vi "Test - Create Property.vi"   [LabVIEW 2020, in "JSON Schema Generator.lvlib"]
uses:
  JSON Schema Generator.lvlib
  <vilib>/addons/_JKI Toolkits/Caraya/classes/Test/Test.lvclass
  <vilib>/Utility/Data Type/Type Definitions/Data Type.ctl
  <vilib>/Utility/Data Type/NI_Data Type.lvlib
  <vilib>/addons/_JKI Toolkits/Caraya/classes/Assert/Assert.lvclass
  <vilib>/JDP Science/JSONtext/JSONtext.lvlib
  <vilib>/addons/_JKI Toolkits/Caraya/classes/Assert/Assert Equal Value_Variant.vi
  f974771b-0b98-47eb-9ce7-aca3fa1358ef.vi
  <vilib>/addons/_JKI Toolkits/Caraya/classes/Assert/Assert Not Error.vi
types:
  T1 = enum16{"Normal Description", "JSON Description"}[]
  T2 = typedef "NI_Data Type.lvlib/Data Type.ctl" = enum8{"Invalid Type", "Void", "I8", "I16", "I32", "I64", "U8", "U16", "U32", "U64", "Single Float", "Double Float", "Extended Float", "Single Complex", "Double Complex", "Extended Complex", "Enum U8", "Enum U16", "Enum U32", "Enum U64", "Single Float With Unit", "Double Float With Unit", "Extended Float With Unit", "Single Complex with Unit", "Double Complex with Unit", "Extended Complex with Unit", "Boolean", "String", "Path", "Picture", "Tag", "Array", "Cluster", "Variant", "LV Variant", "Waveform", "Timestamp", "Digital Waveform", "Digital Data", "ExpressData", "Refnum", "External Data", "VI", "Poly VI", "LabVIEW Class Instance", "Fixed Point", "Set Collection", "Map Collection"}
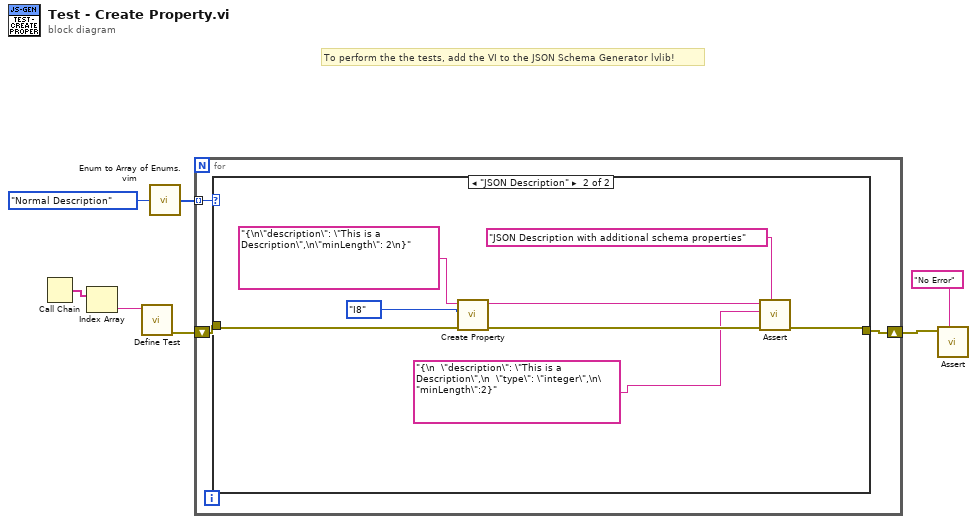
[diagram p0: block diagram]
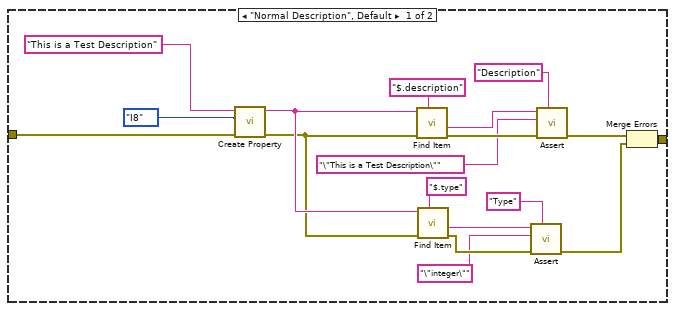
[diagram p2: hidden frame]
diagram:
  # "To perform the the tests, add the VI to the JSON Schema Generator lvlib!"
  n1 = Call Chain() -> (call chain=w7:string[])
  n2 = Index Array(array=w7) -> (element=w6:string)  [unwired: 1 in]
  n3 = call <vilib>:"Define Test.vi"("Label (VI Title)"=w6) -> ("error out"=w5:errorcluster)  [unwired: 9 in, 1 out]
  n4 = call "Enum to Array of Enums.vim"("enum"=enum16{"Normal Description", "JSON Description"}."Normal Description") -> ("array of enums"=w1:T1)
  n5 = for {
    shift-right: [w9] -> w3
    shift-left: w5 -> [w10]
    tunnel: w1 -> [w8] mode=indexing
    n6 = case shown="\"JSON Description\"" w8 {
      tunnel: w10 -> [w28 w32]
      tunnel: [w11 w31] -> w9
      frame "Normal Description", Default {
        n7 = call "Create Property.vi"("error in"=w28, "Labview Type"=Data_Type."I8", "Description"="This is a Test Description") -> ("error out"=w12:errorcluster, "JSON Schema Property out"=w18:string)  [unwired: 7 in]
        n8 = call <vilib>:"Find Item.vi"("$Path or Item Name"="$.description", "error in (no error)"=w12, "JSON"=w18) -> ("error out"=w23:errorcluster, "<JSON>"=w25:string)  [unwired: 5 in, 2 out]
        n9 = call <vilib>:"Find Item.vi"("$Path or Item Name"="$.type", "error in (no error)"=w12, "JSON"=w18) -> ("error out"=w21:errorcluster, "<JSON>"=w20:string)  [unwired: 5 in, 2 out]
        n10 = call-poly <vilib>:"Assert.vi"("Label"="Type", "error in (no error)"=w21, "Actual"="\"integer\"", "Expected"=w20) -> ("error out"=w14:errorcluster)  [unwired: 6 in, 1 out]
        n11 = call-poly <vilib>:"Assert.vi"("Label"="Description", "error in (no error)"=w23, "Actual"="\"This is a Test Description\"", "Expected"=w25) -> ("error out"=w22:errorcluster)  [unwired: 6 in, 1 out]
        n12 = Merge Errors(w22, w14) -> (w11:errorcluster)
      }
      frame "JSON Description" {
        n13 = call "Create Property.vi"("error in"=w32, "Labview Type"=Data_Type."I8", "Description"="{\n\"description\": \"This is a Description\",\n\"minLength\": 2\n}") -> ("error out"=w33:errorcluster, "JSON Schema Property out"=w29:string)  [unwired: 7 in]
        n14 = call-poly <vilib>:"Assert.vi"("Label"="JSON Description with additional schema properties", "error in (no error)"=w33, "Actual"="{\n  \"description\": \"This is a Description\",\n  \"type\": \"integer\",\n\"minLength\":2}", "Expected"=w29) -> ("error out"=w31:errorcluster)  [unwired: 6 in, 1 out]
      }
    }
  }
  n15 = call-poly <vilib>:"Assert.vi"("Label"="No Error", "Not Error?"=w3) -> ()  [unwired: 8 in, 2 out]
